vi "Rio_Theta_Calibration.vi"(8 "Error In":errorcluster) -> (0 "error out":errorcluster)   [LabVIEW 2017]
panel:
  in  "Desired Position":dbl(knob) step=0.9 scale=-90.0..90.0 scale format="%#_6f"
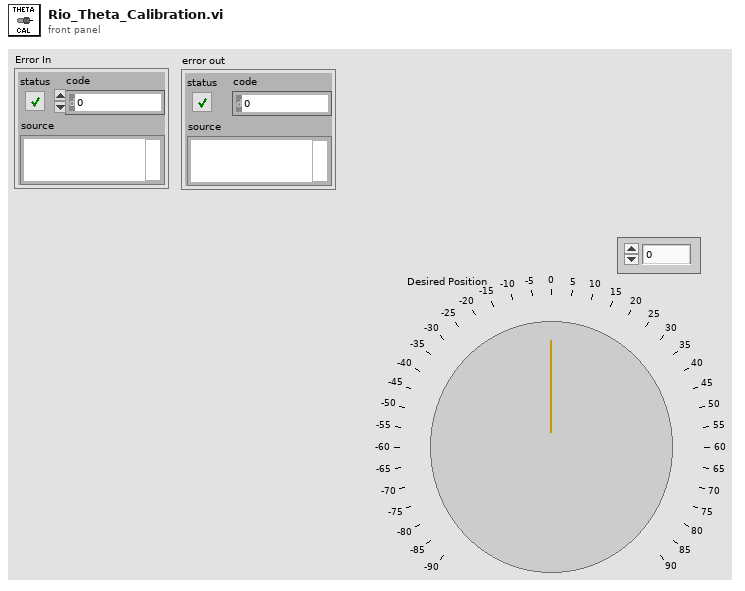
[diagram p1: front panel]
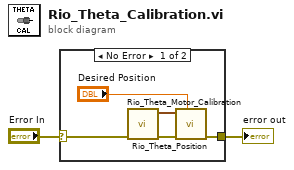
[diagram p0: block diagram]
diagram:
  n1 = case shown="No Error" "Error In" {
    selector: "Error In" -> [w5 w8]
    tunnel: [w7 w8] -> w1
    frame No Error {
      n2 = call "Rio_Theta_Motor_Calibration.vi"("error in (no error)"=w5) -> ("error out"=w6:errorcluster, "Theta Sequence & Position"=w4:cluster{i32, dbl})  [unwired: 9 in]
      n3 = call "Rio_Theta_Position.vi"("Desired Position"="Desired Position", "error in (no error)"=w6, "Theta Sequence & Position"=w4) -> ("error out"=w7:errorcluster)  [unwired: 8 in]
    }
    frame Error {
    }
  }
  "error out" <- w1
